vi "Init.vi"(8 "error in (no error)":errorcluster, 11 "VISA resource in":path=path "C:/Users/zachc/Downloads/tmp") -> (0 "error out":errorcluster, 3 "Data Output File Out":path)   [LabVIEW 2020, in "Waters Patrol UPLC Report Parser.lvlib"]
uses:
  Waters Patrol UPLC Report Parser.lvlib
  Typedefs/Init.vi States.ctl
panel:
  in  "Cancel Btn":bool
  in  "Confirm File Btn":bool
  # "1. Data Output Directory"
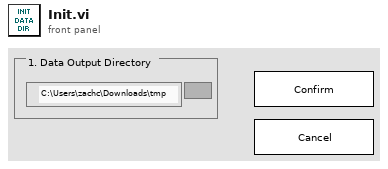
[diagram p1: front panel]
types:
  T1 = typedef "Waters Patrol UPLC Report Parser.lvlib/Init.vi States.ctl" = enum16{"Waiting for connection", "Connecting", "Successful connection", "Failed to connect", "Closing"}
  T2 = enum32{"Invalid", "Standard", "Closed", "Hidden", "Minimized", "Maximized"}
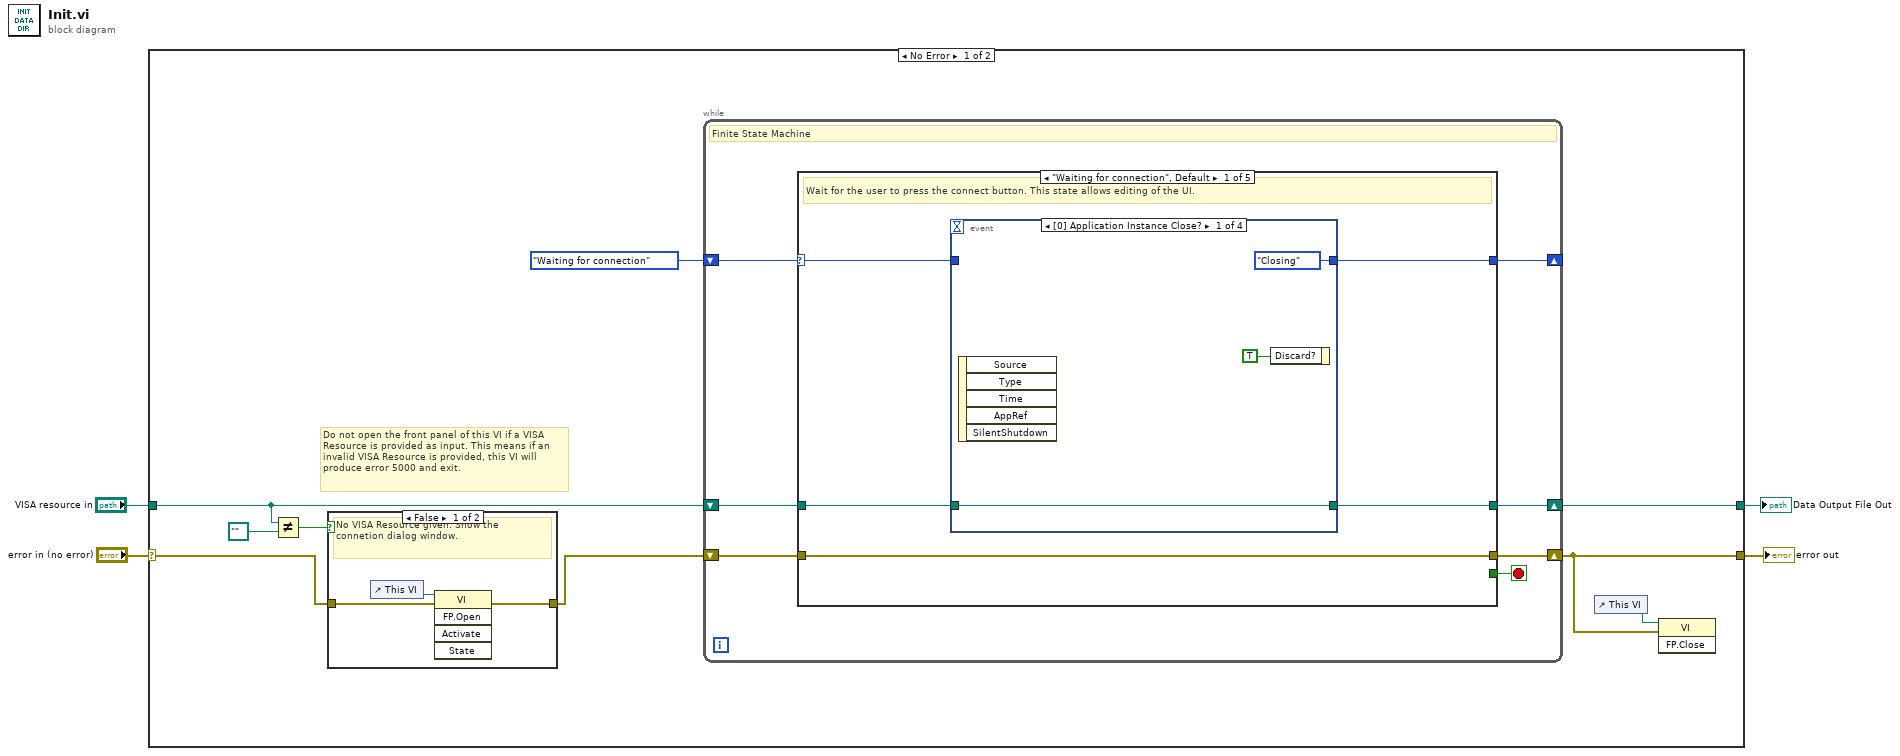
[diagram p0: block diagram]
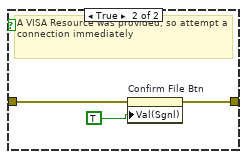
[diagram p2: hidden frame]
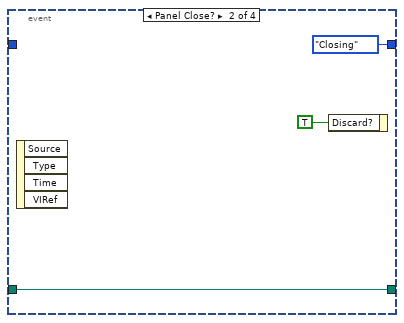
[diagram p3: hidden frame]
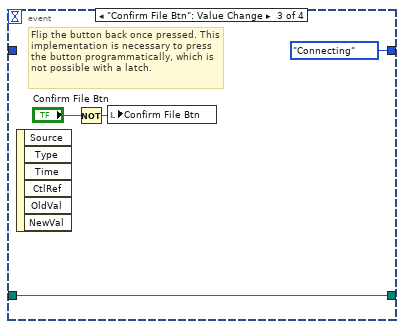
[diagram p4: hidden frame]
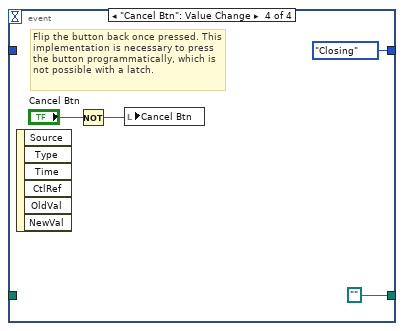
[diagram p5: hidden frame]
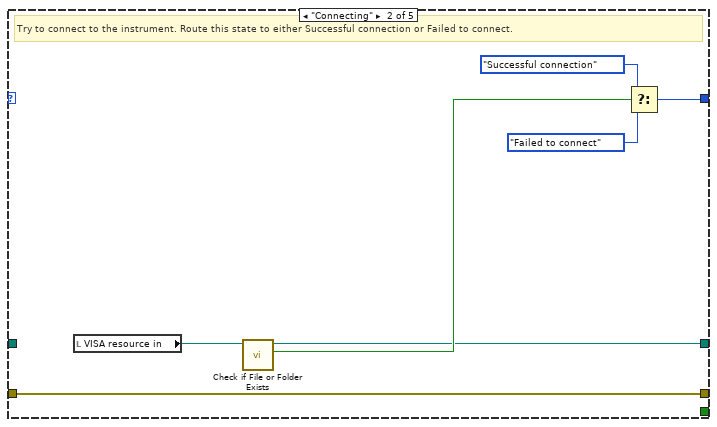
[diagram p6: hidden frame]
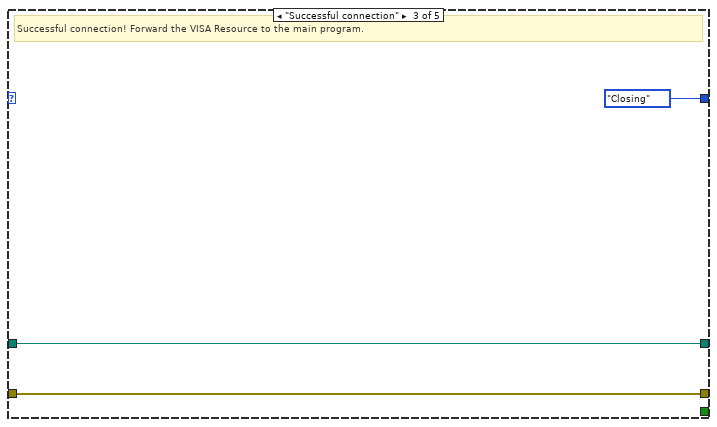
[diagram p7: hidden frame]
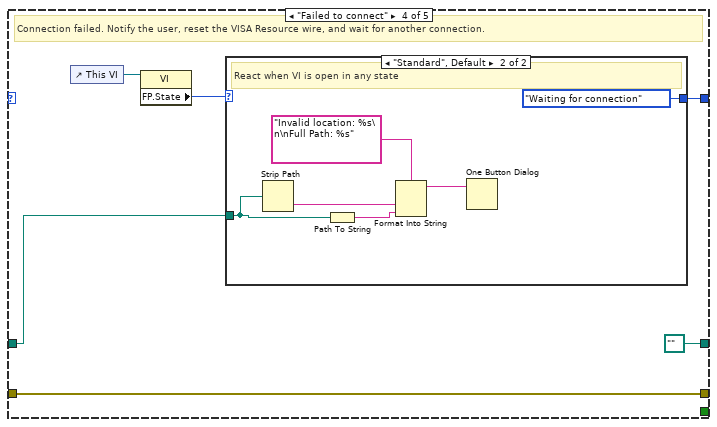
[diagram p8: hidden frame]
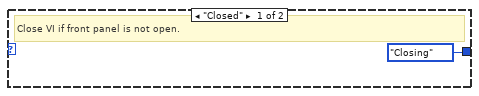
[diagram p9: hidden frame]
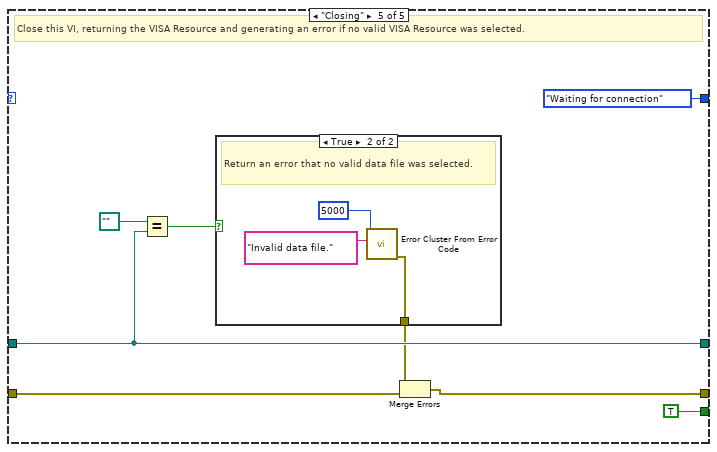
[diagram p10: hidden frame]
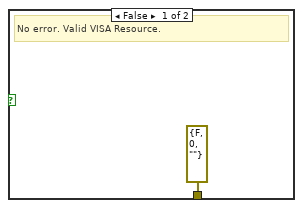
[diagram p11: hidden frame]
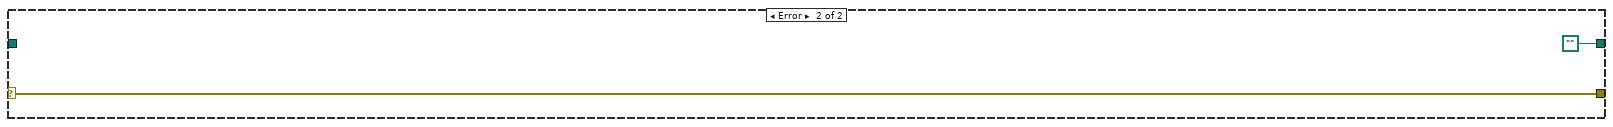
[diagram p12: hidden frame]
diagram:
  n1 = case shown="No Error" "error in (no error)" {
    selector: "error in (no error)" -> [w6 w82]
    tunnel: [w12 path ""] -> w4
    tunnel: [w10 w82] -> w2
    tunnel: "VISA resource in" -> [w7 _]
    frame No Error {
      # "Do not open the front panel of this VI if a VISA Resource is provided as input. This means if an invalid VISA Resource is provided, this VI will produce error 5000 and exit."
      n2 = Not Equal?(x=w7, y=path "" ("x")) -> (x != y?=w9:bool)
      n3 = case shown="False" w9 {
        tunnel: w6 -> [w15 w18]
        tunnel: [w14 w17] -> w5
        frame False {
          # "No VISA Resource given. Show the connetion dialog window."
          n4 = control-ref of="This VI"() -> (w16:refnum<vi>)
          n5 = invoke class="VI" method="FP.Open"(reference=w16, error in=w15) -> (error out=w14:errorcluster)  [unwired: 3 in, 4 out]
        }
        frame True {
          # "A VISA Resource was provided, so attempt a connection immediately"
          n6 = property on="Confirm File Btn" class="Bool (strict)"(error in=w18, "Val(Sgnl)"=TRUE) -> (error out=w17:errorcluster)  [unwired: 1 in, 1 out]
        }
      }
      n7 = while {
        shift-right: [w25] -> _
        shift-left: Init.vi_States."Waiting for connection" -> [w26]
        shift-right: [w23] -> w12
        shift-left: w7 -> [w22]
        shift-right: [w20] -> w10
        shift-left: w5 -> [w21]
        stop <- w24 stop-if-true
        # "Finite State Machine"
        n8 = case shown="\"Waiting for connection\", Default" w26 {
          selector: w26 -> [w31 _ _ _ _]
          tunnel: [w30 w52 Init.vi_States."Closing" w61 Init.vi_States."Waiting for connection"] -> w25
          tunnel: [_ _ _ _ TRUE] -> w24
          tunnel: [w27 w46 w53 path "" ("VISA resource in") w73] -> w23
          tunnel: w22 -> [w28 _ w53 w56 w73]
          tunnel: w21 -> [w29 w49 w54 w59 w69]
          tunnel: [w29 w49 w54 w59 w70] -> w20
          frame "Waiting for connection", Default {
            # "Wait for the user to press the connect button. This state allows editing of the UI."
            n9 = event shown="[0] Application Instance Close?" {
              selector: _ -> [_ _ _ _]
              dyn-events: _ -> [_ _ _ _]
              timeout: _ -> [_ _ _ _]
              tunnel: [Init.vi_States."Closing" Init.vi_States."Closing" Init.vi_States."Connecting" Init.vi_States."Closing"] -> w30
              tunnel: w31 -> [_ _ _ _]
              tunnel: [w32 w35 w38 path ""] -> w27
              tunnel: w28 -> [w32 w35 w38 _]
              event Application Instance Close? {
                n10 = event-data() -> ()  [unwired: 1 in, 5 out]
                n11 = event-data("Discard?"=TRUE) -> ()  [unwired: 1 in, 1 out]
              }
              event Panel Close? {
                n12 = event-data() -> ()  [unwired: 1 in, 4 out]
                n13 = event-data("Discard?"=TRUE) -> ()  [unwired: 1 in, 1 out]
              }
              event "Confirm File Btn": Value Change {
                # "Flip the button back once pressed. This implementation is necessary to press the button programmatically, which is not possible with a latch."
                n14 = event-data() -> ()  [unwired: 1 in, 6 out]
                n15 = Not(x="Confirm File Btn") -> (.not. x?=w39:bool)
                n16 = local write "Confirm File Btn"(w39) -> ()
              }
              event "Cancel Btn": Value Change {
                # "Flip the button back once pressed. This implementation is necessary to press the button programmatically, which is not possible with a latch."
                n17 = event-data() -> ()  [unwired: 1 in, 6 out]
                n18 = Not(x="Cancel Btn") -> (.not. x?=w45:bool)
                n19 = local write "Cancel Btn"(w45) -> ()
              }
            }
          }
          frame "Connecting" {
            # "Try to connect to the instrument. Route this state to either Successful connection or Failed to connect."
            n20 = local read "VISA resource in"() -> (w48:path)
            n21 = call <vilib>:"Check if File or Folder Exists.vi"("path"=w48) -> ("file or folder exists?"=w47:bool, "dup path"=w46:path)  [unwired: 8 in, 1 out]
            n22 = Select(t=Init.vi_States."Successful connection", s=w47, f=Init.vi_States."Failed to connect") -> (s? t:f=w52:T1)
          }
          frame "Successful connection" {
            # "Successful connection! Forward the VISA Resource to the main program."
          }
          frame "Failed to connect" {
            # "Connection failed. Notify the user, reset the VISA Resource wire, and wait for another connection."
            n23 = control-ref of="This VI"() -> (w58:refnum<vi>)
            n24 = property class="VI"(reference=w58) -> ("FP.State"=w57:T2)  [unwired: 1 in, 2 out]
            n25 = case shown="\"Standard\", Default" w57 {
              tunnel: [Init.vi_States."Closing" Init.vi_States."Waiting for connection"] -> w61
              tunnel: w56 -> [_ w65]
              frame "Closed" {
                # "Close VI if front panel is not open."
              }
              frame "Standard", Default {
                # "React when VI is open in any state"
                n26 = Strip Path(path=w65) -> (name=w66:string)  [unwired: 1 out]
                n27 = Path To String(path=w65) -> (string=w64:string)
                n28 = Format Into String(format string="Invalid location: %s\n\nFull Path: %s", w66, w64) -> (resulting string=w63:string)  [unwired: 2 in, 1 out]
                n29 = One Button Dialog(message=w63) -> ()  [unwired: 1 in, 1 out]
              }
            }
          }
          frame "Closing" {
            # "Close this VI, returning the VISA Resource and generating an error if no valid VISA Resource was selected."
            n30 = Equal?(x=path "" ("VISA resource in"), y=w73) -> (x = y?=w72:bool)
            n31 = case shown="True" w72 {
              tunnel: [errorcluster {"status"=FALSE, "code"=0, "source"=""} ("error out") w79] -> w71
              frame False {
                # "No error. Valid VISA Resource."
              }
              frame True {
                # "Return an error that no valid data file was selected."
                n32 = call <vilib>:"Error Cluster From Error Code.vi"("error message (\"\")"="Invalid data file." ("error message (\"\")"), "error code (0)"=5000) -> ("error out"=w79:errorcluster)  [unwired: 7 in]
              }
            }
            n33 = Merge Errors(w71, w69) -> (w70:errorcluster)
          }
        }
      }
      n34 = control-ref of="This VI"() -> (w11:refnum<vi>)
      n35 = invoke class="VI" method="FP.Close"(reference=w11, error in=w10) -> ()  [unwired: 1 in, 3 out]
    }
    frame Error {
    }
  }
  "Data Output File Out" <- w4
  "error out" <- w2
